vi "Login.vi"(4 "Source (\"\")":string, 6 "User ID (\"\")":string, 7 "Bluetooth Password (\"\")":string, 8 "error in (no error)":errorcluster, 9 "Password (\"\")":string, 10 "User Name (\"admin\")":string="admin", 11 "VISA resource name":refnum<visa-resource-name>) -> (0 "error out":errorcluster, 3 "VISA resource name out":refnum<visa-resource-name>)   [LabVIEW 2020, in "Yokogawa GX Series.lvlib"]
doc: "This VI logs in the instrument.\nSpecified user name provides access authority as follows,\n\nAdministrator:\n An administrator has the whole authority.\n\nUser:\n A user has limited authority to use. \n The user can read settings but cannot change settings. \n The user can output the measurement data."
uses:
  <instrlib>/Yokogawa GX Series/Yokogawa GX Series.lvlib
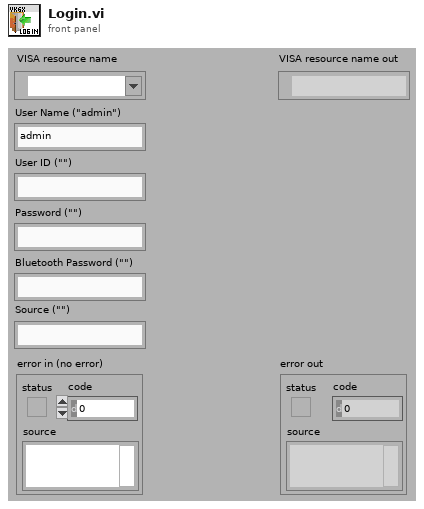
[diagram p1: front panel]
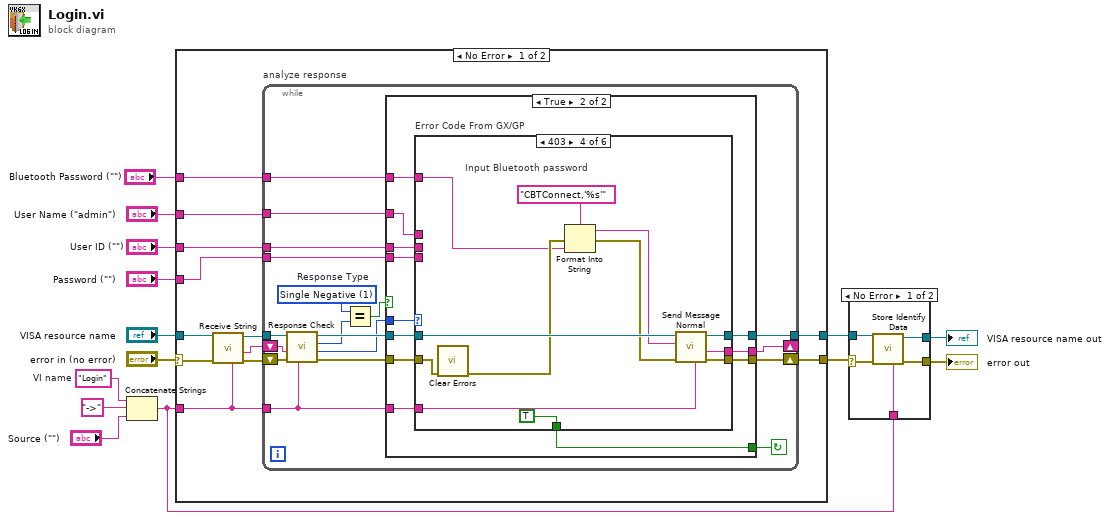
[diagram p0: block diagram]
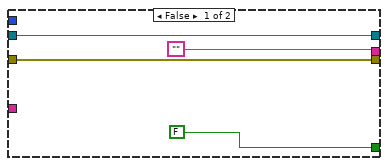
[diagram p3: hidden frame]
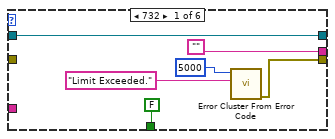
[diagram p4: hidden frame]
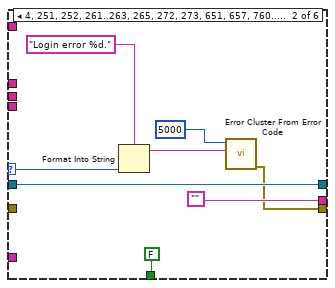
[diagram p5: hidden frame]
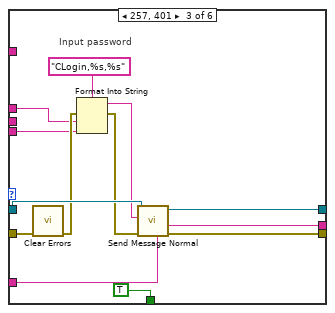
[diagram p6: hidden frame]
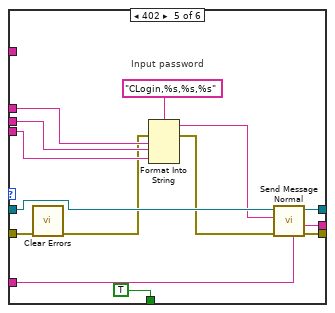
[diagram p7: hidden frame]
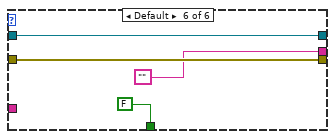
[diagram p8: hidden frame]
diagram:
  w14 = "Login"  # VI name
  n1 = Concatenate Strings(w14, "->", "Source (\"\")") -> (w2:string)
  n2 = case shown="No Error" "error in (no error)" {
    selector: "error in (no error)" -> [w17 w118]
    tunnel: [w26 w119] -> w4
    tunnel: [w25 w118] -> w6
    tunnel: "Password (\"\")" -> [w24 _]
    tunnel: "User Name (\"admin\")" -> [w23 _]
    tunnel: "VISA resource name" -> [w19 w119]
    tunnel: w2 -> [w18 _]
    tunnel: "User ID (\"\")" -> [w16 _]
    tunnel: "Bluetooth Password (\"\")" -> [w15 _]
    frame No Error {
      n3 = call <instrlib>:"Receive String.vi"("Source (\"\")"=w18, "error in (no error)"=w17, "VISA resource name"=w19) -> ("error out"=w22:errorcluster, "Read Buffer"=w21:string, "VISA resource name out"=w20:refnum<visa-resource-name>)  [unwired: 6 in]
      n4 = while "analyze response" {
        shift-left: w22 -> [w39]
        shift-right: [w44] -> w25
        tunnel: w18 -> [w38]
        shift-left: w21 -> [w40]
        shift-right: [w42] -> _
        tunnel: w24 -> [w33]
        tunnel: w23 -> [w34]
        tunnel: w20 -> [w41]
        tunnel: [w43] -> w26
        tunnel: w16 -> [w28]
        tunnel: w15 -> [w27]
        stop <- w30 continue-if-true
        w32 = 1 items=["Affirmative", "Single Negative", "Multiple Negative", "ASCII", "Binary", "End"]  # Response Type
        n5 = call <instrlib>:"Response Check.vi"("Source (\"\")"=w38, "error in (no error)"=w39, "Message In (\"\")"=w40, "VISA resource name"=w41) -> ("error out"=w37:errorcluster, "Internal Error Number"=w31:i32, "Response Type"=w35:i32, "VISA resource name out"=w36:refnum<visa-resource-name>)  [unwired: 4 out]
        n6 = Equal?(x=w32, y=w35) -> (x = y?=w29:bool)
        n7 = case shown="True" w29 {
          tunnel: [w47 w60] -> w44
          tunnel: [w48 w59] -> w43
          tunnel: ["" w58] -> w42
          tunnel: w38 -> [_ w57]
          tunnel: w37 -> [w47 w56]
          tunnel: w36 -> [w48 w55]
          tunnel: w34 -> [_ w54]
          tunnel: w33 -> [_ w53]
          tunnel: w31 -> [_ w52]
          tunnel: [FALSE w51] -> w30
          tunnel: w28 -> [_ w50]
          tunnel: w27 -> [_ w49]
          frame False {
          }
          frame True {
            n8 = case "Error Code From GX/GP" shown="403" w52 {
              selector: w52 -> [_ w70 _ _ _ _]
              tunnel: w53 -> [_ _ w79 _ w105 _]
              tunnel: w54 -> [_ _ w80 _ w107 _]
              tunnel: w57 -> [_ _ w83 w95 w110 _]
              tunnel: w55 -> [w66 w74 w85 w97 w104 w117]
              tunnel: w56 -> [_ _ w87 w99 w113 w116]
              tunnel: [w63 w68 w75 w89 w109 w116] -> w60
              tunnel: [w66 w74 w84 w96 w111 w117] -> w59
              tunnel: ["" "" w76 w90 w108 ""] -> w58
              tunnel: [FALSE FALSE TRUE TRUE TRUE FALSE] -> w51
              tunnel: w50 -> [_ _ _ _ w106 _]
              tunnel: w49 -> [_ _ _ w88 _ _]
              frame 732 {
                n9 = call <vilib>:"Error Cluster From Error Code.vi"("error message (\"\")"="Limit Exceeded.", "error code (0)"=5000) -> ("error out"=w63:errorcluster)  [unwired: 7 in]
              }
              frame 4, 251, 252, 261..263, 265, 272, 273, 651, 657, 760..775 {
                n10 = Format Into String(format string="Login error %d.", w70) -> (resulting string=w69:string)  [unwired: 2 in, 1 out]
                n11 = call <vilib>:"Error Cluster From Error Code.vi"("error message (\"\")"=w69, "error code (0)"=5000) -> ("error out"=w68:errorcluster)  [unwired: 7 in]
              }
              frame 257, 401 {
                # "Input password"
                n12 = call <vilib>:"Clear Errors.vi"("error in (no error)"=w87) -> ("error out"=w81:errorcluster)  [unwired: 1 in, 5 out]
                n13 = Format Into String(format string="CLogin,%s,%s", error in=w81, w80, w79) -> (resulting string=w78:string, error out=w77:errorcluster)  [unwired: 1 in]
                n14 = call <instrlib>:"Send Message Normal.vi"("Source (\"\")"=w83, "error in (no error)"=w77, "Send Message (\"\")"=w78, "VISA resource name"=w85) -> ("error out"=w75:errorcluster, "Read Buffer"=w76:string, "VISA resource name out"=w84:refnum<visa-resource-name>)  [unwired: 5 in]
              }
              frame 403 {
                # "Input Bluetooth password"
                n15 = call <vilib>:"Clear Errors.vi"("error in (no error)"=w99) -> ("error out"=w93:errorcluster)  [unwired: 1 in, 5 out]
                n16 = Format Into String(format string="CBTConnect,'%s'", error in=w93, w88) -> (resulting string=w92:string, error out=w91:errorcluster)  [unwired: 1 in]
                n17 = call <instrlib>:"Send Message Normal.vi"("Source (\"\")"=w95, "error in (no error)"=w91, "Send Message (\"\")"=w92, "VISA resource name"=w97) -> ("error out"=w89:errorcluster, "Read Buffer"=w90:string, "VISA resource name out"=w96:refnum<visa-resource-name>)  [unwired: 5 in]
              }
              frame 402 {
                # "Input password"
                n18 = call <vilib>:"Clear Errors.vi"("error in (no error)"=w113) -> ("error out"=w103:errorcluster)  [unwired: 1 in, 5 out]
                n19 = Format Into String(format string="CLogin,%s,%s,%s", error in=w103, w107, w106, w105) -> (resulting string=w101:string, error out=w102:errorcluster)  [unwired: 1 in]
                n20 = call <instrlib>:"Send Message Normal.vi"("Source (\"\")"=w110, "error in (no error)"=w102, "Send Message (\"\")"=w101, "VISA resource name"=w104) -> ("error out"=w109:errorcluster, "Read Buffer"=w108:string, "VISA resource name out"=w111:refnum<visa-resource-name>)  [unwired: 5 in]
              }
              frame Default {
              }
            }
          }
        }
      }
    }
    frame Error {
    }
  }
  n21 = case shown="No Error" w6 {
    selector: w6 -> [w124 w125]
    tunnel: [w123 w125] -> w5
    tunnel: w4 -> [w122 w126]
    tunnel: [w121 w126] -> w3
    tunnel: w2 -> [w120 _]
    frame No Error {
      n22 = call <instrlib>:"Store Identify Data.vi"("Source (\"\")"=w120, "error in (no error)"=w124, "VISA resource name"=w122) -> ("error out"=w123:errorcluster, "VISA resource name out"=w121:refnum<visa-resource-name>)  [unwired: 7 in]
    }
    frame Error {
    }
  }
  "error out" <- w5
  "VISA resource name out" <- w3
